vi "Remove Plugsin from Map.vi"(10 "plugin_info":T4[](array[typedef]) {"Node Status"."Monitor Doubles"."4" format="%#_9g"; "Node Status"."Monitor Doubles"."3" format="%#_9g"; "Node Status"."Monitor Doubles"."2" format="%#_9g"; "Node Status"."Monitor Doubles"."1" format="%#_9g"; "Node Status"."Timing Statistics (us)"."Period"."Avg" format="%_6g"}, 11 "Plugin Connection Map in":T1 {"Plugin Connections"."Plugin Info"."Node Status"."Monitor Doubles"."4" format="%#_9g"; "Plugin Connections"."Plugin Info"."Node Status"."Monitor Doubles"."3" format="%#_9g"; "Plugin Connections"."Plugin Info"."Node Status"."Monitor Doubles"."2" format="%#_9g"; "Plugin Connections"."Plugin Info"."Node Status"."Monitor Doubles"."1" format="%#_9g"}) -> (3 "Plugin Connection Map out":T1 {"Plugin Connections"."Plugin Info"."Node Status"."Monitor Doubles"."4" format="%#_9g"; "Plugin Connections"."Plugin Info"."Node Status"."Monitor Doubles"."3" format="%#_9g"; "Plugin Connections"."Plugin Info"."Node Status"."Monitor Doubles"."2" format="%#_9g"; "Plugin Connections"."Plugin Info"."Node Status"."Monitor Doubles"."1" format="%#_9g"})   [LabVIEW 2021, in "CIF_UI.lvclass"]
uses:
  CIF_UI.lvclass
  CIF_UI.lvclass/CIF_UI.ctl
  <vilib>/gRPC/LabVIEW gRPC Library/grpc-lvsupport-release.lvlib
  Typedef/Version.ctl
  CIFCore/Common/Typedef/Plugin State.ctl
  CIFCore/Common/CIFCoreCommon.lvlib
  CIFCore/Common/Typedef/Timing Stats Base.ctl
  CIFCore/Common/Typedef/Timing Statistics.ctl
  CIFCore/Common/Typedef/FIFO Statistics.ctl
  CIFCore/Common/Typedef/Simple Error.ctl
  CIFCore/Common/Typedef/Monitor Doubles.ctl
  CIFCore/Common/Typedef/Monitor U64.ctl
  CIFCore/Common/Typedef/Monitor I64.ctl
  CIFCore/Common/Typedef/gRPC Reported Plugin Status.ctl
  Typedef/PluginInfo.ctl
  <vilib>/gRPC/LabVIEW gRPC Library/Shared/grpcId.ctl
  Typedef/Plugin Connections.ctl
  Typedef/Plugin Connection Map.ctl
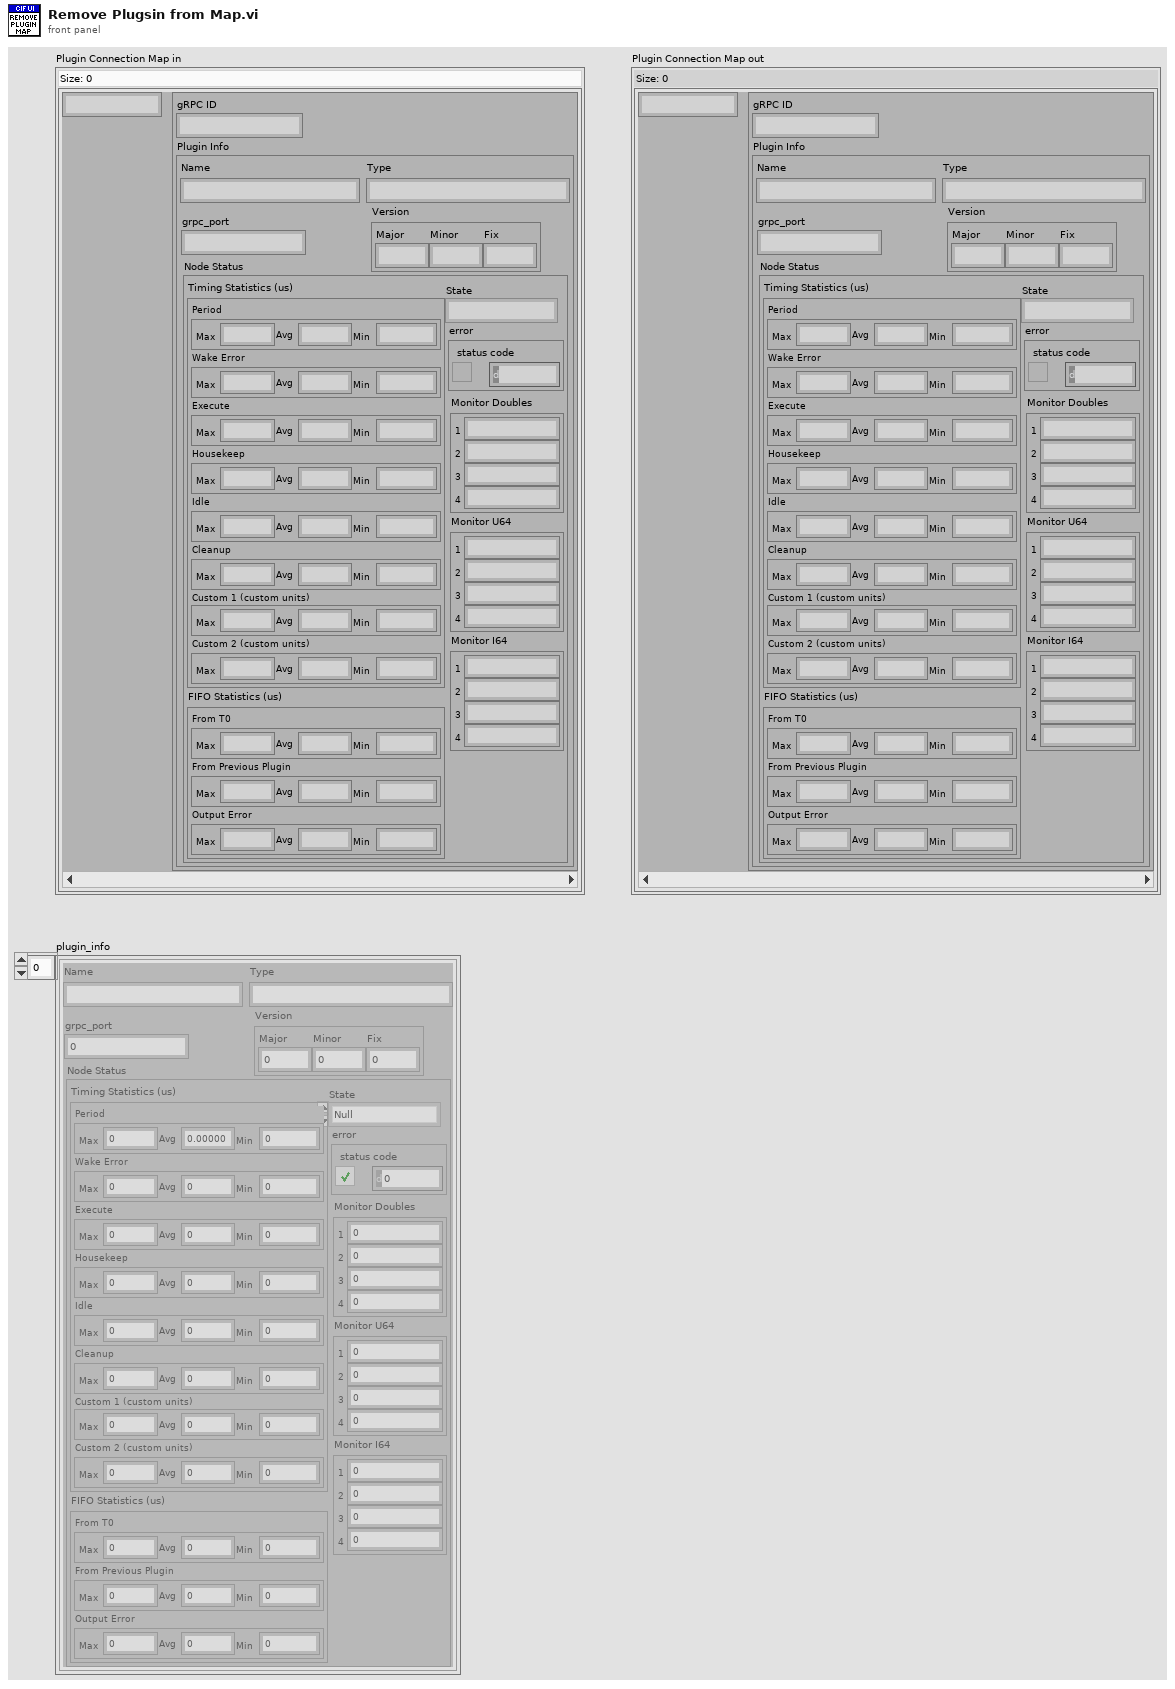
[diagram p1: front panel]
types:
  T1 = typedef "CIF_UI.lvclass/Plugin Connection Map.ctl" = map{string, T2}
  T2 = typedef "CIF_UI.lvclass/Plugin Connections.ctl" = cluster{"gRPC ID":T3, "Plugin Info":T4}
  T3 = typedef "grpc-lvsupport-release.lvlib/grpcId.ctl" = u64
  T4 = typedef "CIF_UI.lvclass/PluginInfo.ctl" = cluster{"Name":string, "Type":string, "grpc_port":i32, "Version":T5, "Node Status":T6}
  T5 = typedef "CIF_UI.lvclass/Version.ctl" = cluster{"Major":i32, "Minor":i32, "Fix":i32}
  T6 = typedef "CIFCoreCommon.lvlib/gRPC Reported Plugin Status.ctl" = cluster{"State":T7, "Timing Statistics (us)":T8, "FIFO Statistics (us)":T10, "error":T11, "Monitor Doubles":T12, "Monitor U64":T13, "Monitor I64":T14}
  T7 = typedef "CIFCoreCommon.lvlib/Plugin State.ctl" = enum32{"Null", "Creating", "Listening", "Running", "CleaningUp", "Destroying"}
  T8 = typedef "CIFCoreCommon.lvlib/Timing Statistics.ctl" = cluster{"Period":T9, "Wake Error":T9, "Execute":T9, "Housekeep":T9, "Idle":T9, "Cleanup":T9, "Custom 1 (custom units)":T9, "Custom 2 (custom units)":T9}
  T9 = typedef "CIFCoreCommon.lvlib/Timing Stats Base.ctl" = cluster{"Max":i64, "Avg":dbl, "Min":i64}
  T10 = typedef "CIFCoreCommon.lvlib/FIFO Statistics.ctl" = cluster{"From T0":T9, "From Previous Plugin":T9, "Output Error":T9}
  T11 = typedef "CIFCoreCommon.lvlib/Simple Error.ctl" = cluster{"status":bool, "code":i32}
  T12 = typedef "CIFCoreCommon.lvlib/Monitor Doubles.ctl" = cluster{"1":dbl, "2":dbl, "3":dbl, "4":dbl}
  T13 = typedef "CIFCoreCommon.lvlib/Monitor U64.ctl" = cluster{"1":u64, "2":u64, "3":u64, "4":u64}
  T14 = typedef "CIFCoreCommon.lvlib/Monitor I64.ctl" = cluster{"1":i64, "2":i64, "3":i64, "4":i64}
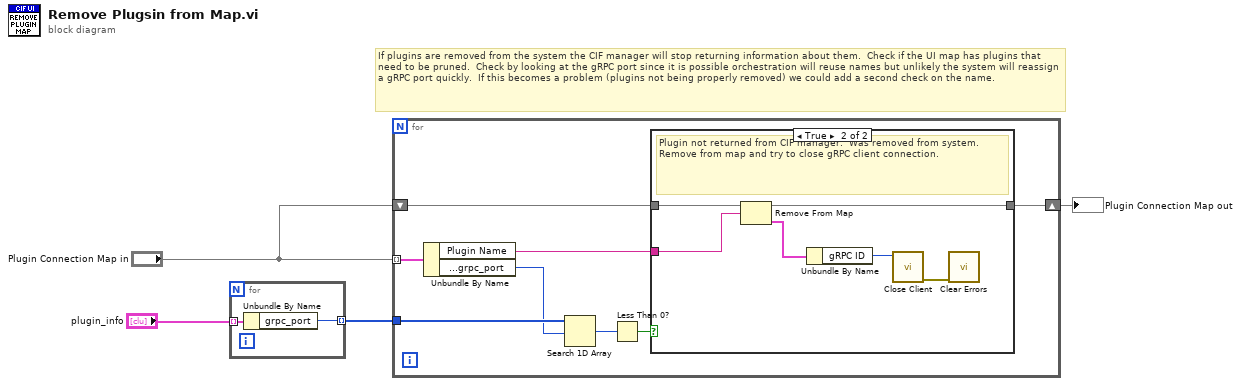
[diagram p0: block diagram]
diagram:
  # "If plugins are removed from the system the CIF manager will stop returning information about them.  Check if the UI map has plugins that need to be pruned.  Check by looking at the gRPC port since it is possible orchestration will reuse names but unlikely the system will reassign a gRPC port quickly.  If this becomes a problem (plugins not being properly removed) we could add a second check on the name."
  n1 = for {
    tunnel: "plugin_info" -> [w6] mode=indexing
    tunnel: [w5] -> w3 mode=indexing
    n2 = Unbundle By Name(w6) -> ("grpc_port"=w5:i32)
  }
  n3 = for {
    tunnel: "Plugin Connection Map in" -> [w14] mode=indexing
    tunnel: w3 -> [w13]
    shift-right: [w7] -> w1
    shift-left: "Plugin Connection Map in" -> [w10]
    n4 = Unbundle By Name(w14) -> ("Plugin Name"=w9:string, "Plugin Connections.Plugin Info.grpc_port"=w12:i32)
    n5 = Search 1D Array(1D array=w13, element=w12) -> (index of element=w11:i32)  [unwired: 1 in]
    n6 = Less Than 0?(x=w11) -> (x < 0?=w8:bool)
    n7 = case shown="True" w8 {
      tunnel: w10 -> [w15 w21]
      tunnel: w9 -> [_ w20]
      tunnel: [w15 w16] -> w7
      frame False {
      }
      frame True {
        # "Plugin not returned from CIF manager.  Was removed from system.  Remove from map and try to close gRPC client connection."
        n8 = Remove From Map(10:w20, 11:w21) -> (1:w19:T2, 3:w16:T1)  [unwired: 1 out]
        n9 = Unbundle By Name(w19) -> ("gRPC ID"=w18:T3)
        n10 = call <vilib>:"Close Client.vi"("ClientID in"=w18) -> ("error out"=w17:errorcluster)  [unwired: 10 in]
        n11 = call <vilib>:"Clear Errors.vi"("error in (no error)"=w17) -> ()  [unwired: 5 in, 2 out]
      }
    }
  }
  "Plugin Connection Map out" <- w1
